vi "IVStepCalculate.vi"(7 "V(0)/I(1)":i32, 9 "End":dbl[](array[numeric]), 10 "Interval":dbl[](array[numeric]), 11 "Start":dbl format="%#_13g") -> (3 "mV/uA":dbl[](array[numeric]))   [LabVIEW 2016]
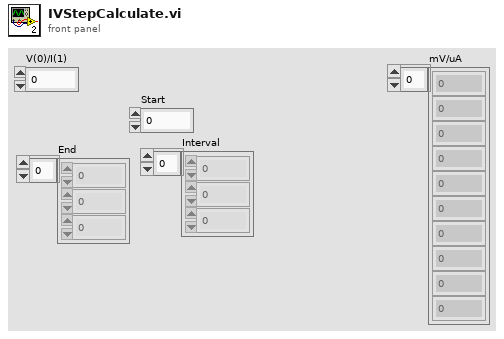
[diagram p1: front panel]
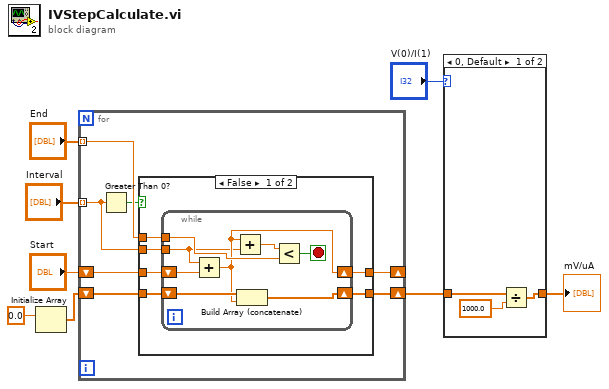
[diagram p0: block diagram]
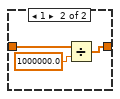
[diagram p2: hidden frame]
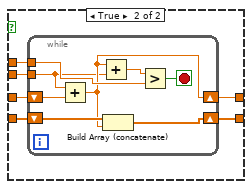
[diagram p3: hidden frame]
diagram:
  n1 = Initialize Array(0.0 ("element")) -> (w4:dbl[])  [unwired: 1 in]
  n2 = for {
    tunnel: "Interval" -> [w10] mode=indexing
    tunnel: "End" -> [w12] mode=indexing
    shift-right: [w13] -> _
    shift-left: "Start" -> [w11]
    shift-right: [w14] -> w3
    shift-left: w4 -> [w15]
    n3 = Greater Than 0?(x=w10) -> (x > 0?=w9:bool)
    n4 = case shown="False" w9 {
      tunnel: w10 -> [w20 w35]
      tunnel: w11 -> [w19 w34]
      tunnel: w15 -> [w18 w33]
      tunnel: [w16 w32] -> w14
      tunnel: [w17 w31] -> w13
      tunnel: w12 -> [w21 w30]
      frame False {
        n5 = while {
          tunnel: w20 -> [w22]
          shift-right: [w24] -> w17
          shift-left: w19 -> [w29]
          shift-right: [w26] -> w16
          shift-left: w18 -> [w27]
          tunnel: w21 -> [w25]
          stop <- w28 stop-if-true
          n6 = Add(x=w22, y=w29) -> (x+y=w24:dbl)
          n7 = Add(x=w24, y=w22) -> (x+y=w23:dbl)
          n8 = Build Array (concatenate)(w27, w24) -> (w26:dbl[])
          n9 = Less?(x=w23, y=w25) -> (x < y?=w28:bool)
        }
      }
      frame True {
        n10 = while {
          tunnel: w35 -> [w36]
          shift-right: [w38] -> w31
          shift-left: w34 -> [w43]
          shift-right: [w40] -> w32
          shift-left: w33 -> [w41]
          tunnel: w30 -> [w39]
          stop <- w42 stop-if-true
          n11 = Add(x=w36, y=w43) -> (x+y=w38:dbl)
          n12 = Add(x=w38, y=w36) -> (x+y=w37:dbl)
          n13 = Build Array (concatenate)(w41, w38) -> (w40:dbl[])
          n14 = Greater?(x=w37, y=w39) -> (0:w42:bool)
        }
      }
    }
  }
  n15 = case shown="0, Default" "V(0)/I(1)" {
    tunnel: w3 -> [w46 w49]
    tunnel: [w45 w47] -> w2
    frame 0, Default {
      n16 = Divide(x=w46, y=1000.0) -> (x/y=w45:dbl[])
    }
    frame 1 {
      n17 = Divide(x=w49, y=1000000.0) -> (x/y=w47:dbl[])
    }
  }
  "mV/uA" <- w2
